vi "Kalman_Estimator_Sepios.vi"(8 "error in":errorcluster) -> (0 "error out":errorcluster)   [LabVIEW 2013]
uses:
  Controls/EKF_Settings.ctl
  Controls/Estimated Position.ctl
  myRIO/Sensors/IMU/IMU_Data_Type_Def.ctl
  <vilib>/imath/engines/lvmath2/RunTimeEngine/ErrorHandling/NIMS_Finalize Error.vi
  <vilib>/imath/engines/lvmath2/RunTimeEngine/BuiltInFunctions/transpose/NIMS_transpose(GV).vi
  <instcachedir>/0/NIMS_transpose(GV)_1D76875BF542458FA31D2D0CC3E998C0.lvgen/NIMS_transpose(GV)_1D76875BF542458FA31D2D0CC3E998C0_000.vi
  <vilib>/imath/engines/lvmath2/RunTimeEngine/NodeEndStatement/NIMS_NodeEndStatement_Output.vi
  <instcachedir>/0/NIMS_NodeEndStatement_Output_53EC0D466D134D7ABD903AC30B43404B.lvgen/NIMS_NodeEndStatement_Output_53EC0D466D134D7ABD903AC30B43404B_003.vi
  <vilib>/imath/engines/lvmath2/RunTimeEngine/IndexRead/NIMS M(R2,S).vi
  <instcachedir>/0/NIMS M(R2,S)_56813DCFDD5A484292D2195AF15D2BF5.lvgen/NIMS M(R2,S)_56813DCFDD5A484292D2195AF15D2BF5_000.vi
  LabVIEW Data/MathScriptVIs/MCStatic_31886544032_2b8e9d258c2bd0716154cc05b7ba0fc2.vi
  <instcachedir>/0/MCStatic_31886544032_2b8e9d258c2bd0716154cc05b7ba0fc2_7C617B4E47594FCE907F90DAAB7145D8.lvgen/MCStatic_31886544032_2b8e9d258c2bd0716154cc05b7ba0fc2_7C617B4E47594FCE907F90DAAB7145D8_001.vi
  <vilib>/imathl/engines/lvmath/Functions/Error Handling/Create Error.vi
  <vilib>/Analysis/Matrix/Numeric/Conversions/Array To Matrix - RA.vi
  <vilib>/imath/engines/lvmath2/RunTimeEngine/Managers/WorkSpace/UID Generator.vi
  <vilib>/Analysis/Matrix/Numeric/Conversions/Matrix To Array - RM.vi
  <vilib>/imath/engines/lvmath2/RunTimeEngine/Managers/SymbolTable/Clear UID.vi
  <instcachedir>/0/NIMS_NodeEndStatement_Output_53EC0D466D134D7ABD903AC30B43404B.lvgen/NIMS_NodeEndStatement_Output_53EC0D466D134D7ABD903AC30B43404B_005.vi
  <instcachedir>/0/NIMS_NodeEndStatement_Output_53EC0D466D134D7ABD903AC30B43404B.lvgen/NIMS_NodeEndStatement_Output_53EC0D466D134D7ABD903AC30B43404B_002.vi
  <vilib>/imath/engines/lvmath2/RunTimeEngine/IndexRead/NIMS M($,S).vi
  <instcachedir>/0/NIMS M($,S)_3E5749BBB62E49528D4765A77F1F6D98.lvgen/NIMS M($,S)_3E5749BBB62E49528D4765A77F1F6D98_000.vi
  LabVIEW Data/MathScriptVIs/MCStatic_31886544032_64f10158a8bf12996c49fb21306ba776.vi
  <instcachedir>/0/MCStatic_31886544032_64f10158a8bf12996c49fb21306ba776_B5FBB23362534537B3F8C988888AB429.lvgen/MCStatic_31886544032_64f10158a8bf12996c49fb21306ba776_B5FBB23362534537B3F8C988888AB429_001.vi
  <vilib>/imath/engines/lvmath2/RunTimeEngine/RunTimeType/NIMS_RunTimeType_From StrictType (excl LVString).vi
  <instcachedir>/0/NIMS_RunTimeType_From StrictType (excl LVString)_4DEE718D6EB74582AA20236969C084FC.lvgen/NIMS_RunTimeType_From StrictType (excl LVString)_4DEE718D6EB74582AA20236969C084FC_000.vi
  <vilib>/imath/engines/lvmath2/RunTimeEngine/LocalVariableDefStatement/MC_LocalVariableDefStatement_Display.vi
  <vilib>/imath/engines/lvmath2/RunTimeEngine/ErrorHandling/NIMS_Create Error From Enums.vi
  <instcachedir>/0/MCStatic_31886544032_64f10158a8bf12996c49fb21306ba776_B5FBB23362534537B3F8C988888AB429.lvgen/MCStatic_31886544032_64f10158a8bf12996c49fb21306ba776_B5FBB23362534537B3F8C988888AB429_000.vi
  Kalman_Estimator_Matlab_Sepios/matlab_tools/quaternion/q_q2rpy.m
  Kalman_Estimator_Matlab_Sepios/matlab_tools/kalman_filter/extended_kalman_filter_process_wpressure_offset_compass_exinit.m
  Kalman_Estimator_Matlab_Sepios/matlab_tools/quaternion/q_min.m
  Kalman_Estimator_Matlab_Sepios/matlab_tools/quaternion/q_mul.m
  Kalman_Estimator_Matlab_Sepios/matlab_tools/quaternion/q_norm.m
  Kalman_Estimator_Matlab_Sepios/matlab_tools/quaternion/q_q2R.m
  Kalman_Estimator_Matlab_Sepios/matlab_tools/quaternion/q_w2Omega.m
  Kalman_Estimator_Matlab_Sepios/matlab_tools/quaternion/skewOp.m
  <vilib>/Analysis/Matrix/NI_Matrix.lvlib
  <vilib>/imath/engines/lvmath2/RunTimeEngine/Managers/SymbolTable/NIMS_WorkSpace.lvlib
panel:
  # "quaternion"
  # "p body position"
  # "v body velocity"
  # "gyro bias"
  # "accel bias"
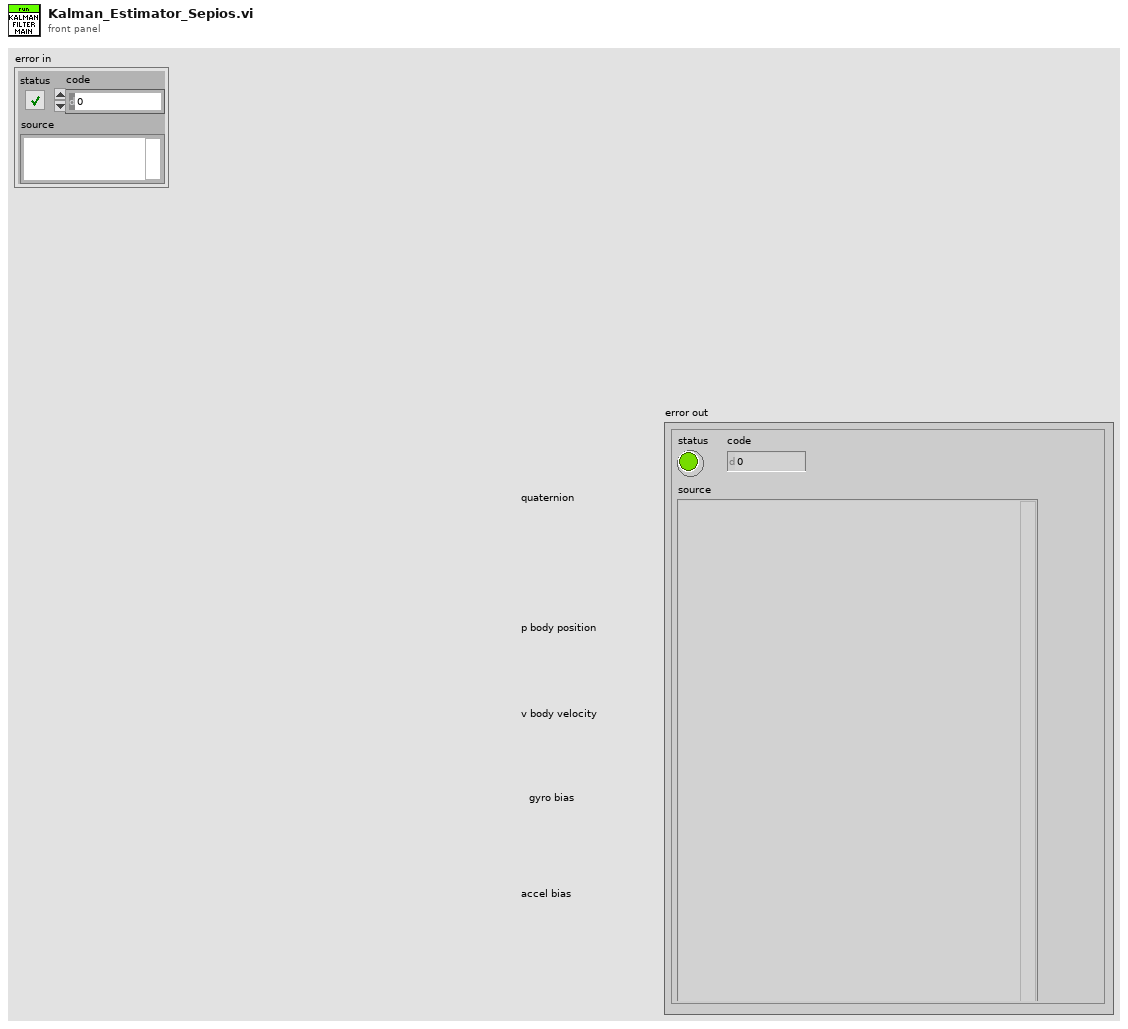
[diagram p1: front panel]
types:
  T1 = typedef "Estimated Position.ctl" = cluster{"X":dbl, "Y":dbl, "Z":dbl, "V_X":dbl, "V_Y":dbl, "V_Z":dbl}
  T2 = typedef "EKF_Settings.ctl" = cluster{"Gravity constant":dbl, "Filter Version":enum16{"IMU Only", "IMU & Pressure", "IMU, Pressure, Compass"}, "Initial Biases":cluster{"Gyro_Bias_nit_x":dbl, "Gyro_Bias_init_y":dbl, "Gyro_Bias_init_z":dbl, "Acc_Bias_init_x":dbl, "Acc_Bias_init_y":dbl, "Acc_Bias_init_z":dbl}, "Use Compass on initialisation":bool, "Initial Biases Covariances":cluster{"Initial_covariance_Gyro_Bias":dbl, "Initial_covariance_Acc_Bias":dbl}, "Magnetic-Field-Vector [utesla]":cluster{"Magf_N_x":dbl, "Magf_N_y":dbl, "Magf_N_z":dbl}, "IMU_Sigmas":cluster{"Sigma_w":dbl, "Sigma_wb":dbl, "Sigma_a":dbl, "Sigma_ab":dbl, "Sigma_m":dbl}, "Measurement Sigmas":cluster{"Sigma_v":dbl, "Sigma_depth":dbl}}
  T3 = typedef "NI_Matrix.lvlib/RealMatrix.ctl" = dbl[][]
  T4 = typedef "IMU_Data_Type_Def.ctl" = cluster{timestamp, "X_Gyro_Out":dbl, "Y_Gyro_Out":dbl, "Z_Gyro_Out":dbl, "X_Accl_Out":dbl, "Y_Accl_Out":dbl, "Z_Accl_Out":dbl, "X_Magn_Out":dbl, "Y_Magn_Out":dbl, "Z_Magn_Out":dbl, "Temp_Out":dbl, "Barom_Out":dbl}
  T5 = enum16{"IMU Only", "IMU & Pressure", "IMU, Pressure, Compass"}
  T6 = cluster{"Magf_N_x":dbl, "Magf_N_y":dbl, "Magf_N_z":dbl}
  T7 = cluster{"Sigma_w":dbl, "Sigma_wb":dbl, "Sigma_a":dbl, "Sigma_ab":dbl, "Sigma_m":dbl}
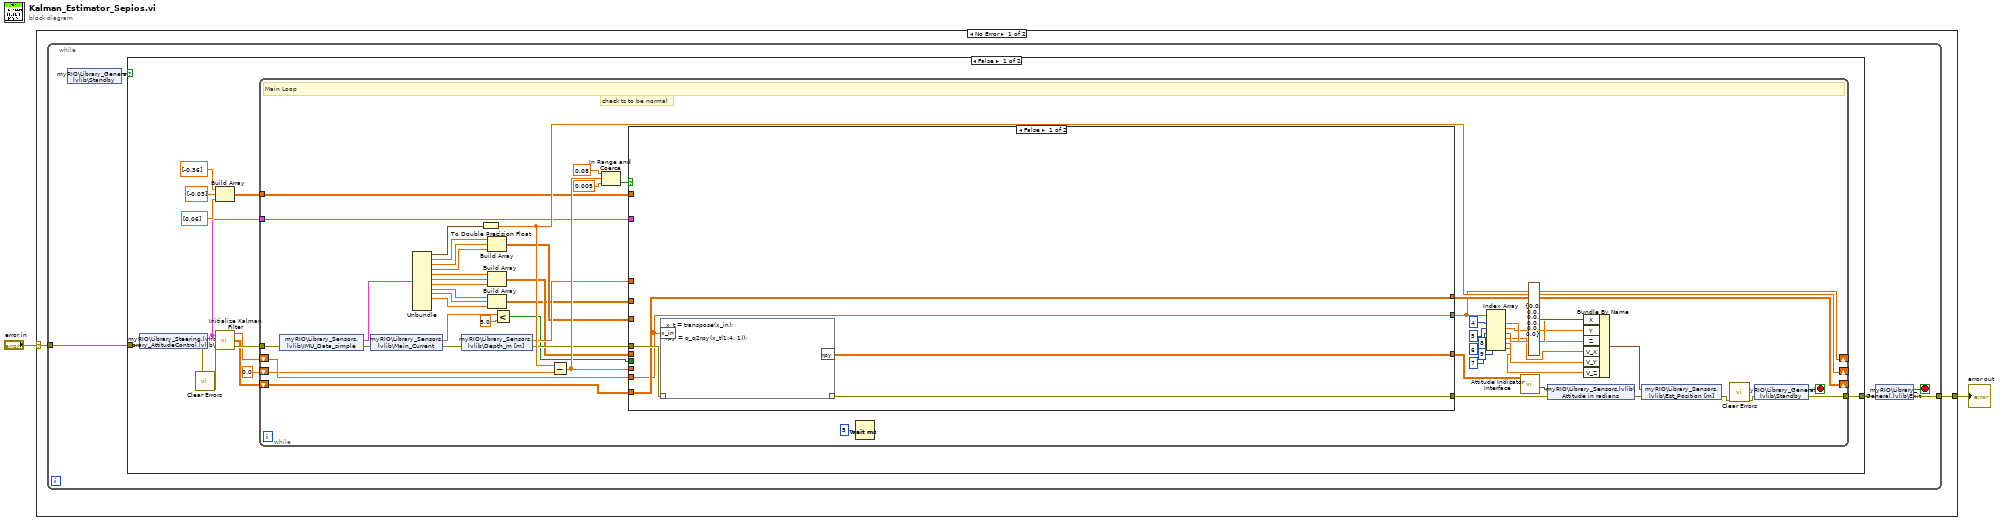
[diagram p0: block diagram]
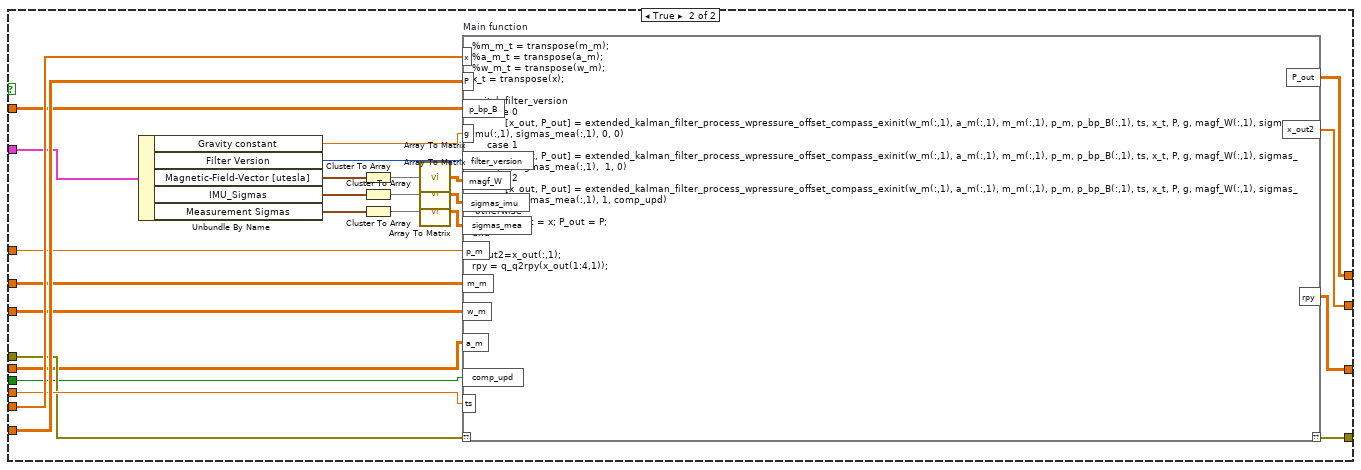
[diagram p2: hidden frame]
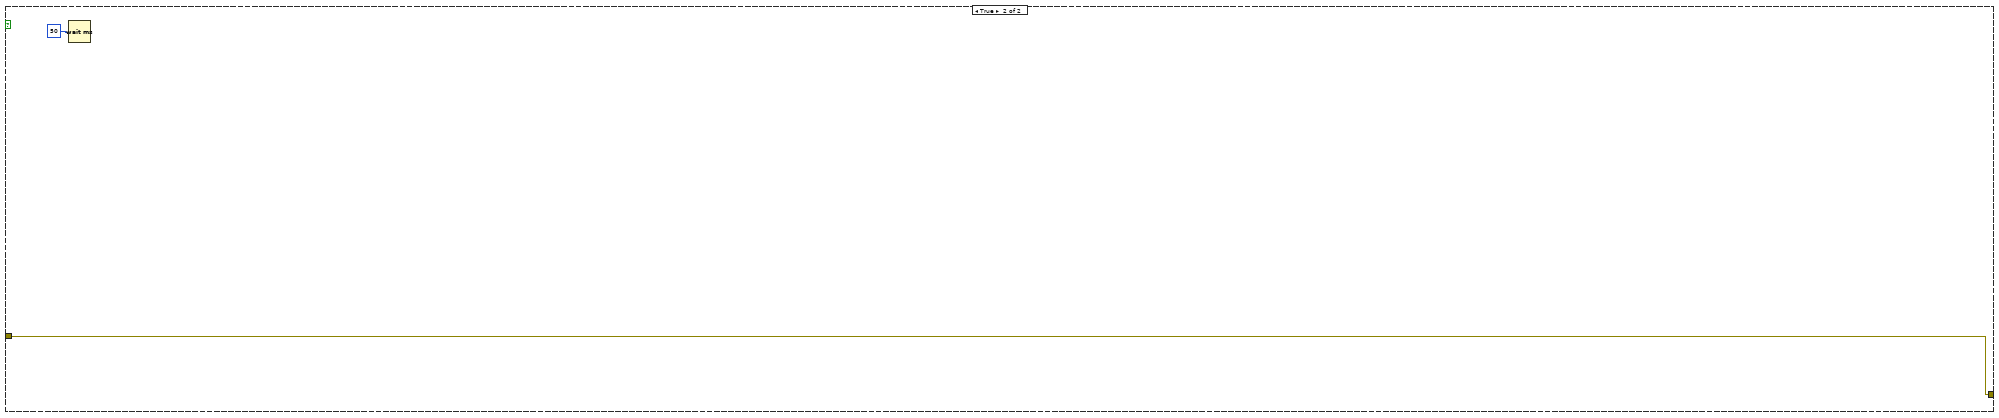
[diagram p3: hidden frame]
diagram:
  n1 = case shown="No Error" "error in" {
    selector: "error in" -> [w3 w646]
    tunnel: [w4 w646] -> w2
    frame No Error {
      n2 = while {
        tunnel: [w5] -> w4
        tunnel: w3 -> [w8]
        stop <- w9 stop-if-true
        n3 = shared-variable "myRIO\\Library_General.lvlib\\Standby"() -> (w7:bool)  [unwired: 1 in, 1 out]
        n4 = case shown="False" w7 {
          tunnel: [w22 w644] -> w6
          tunnel: w8 -> [w18 w644]
          frame False {
            n5 = shared-variable "myRIO\\Library_Steering.lvlib\\Library_AttitudeControl.lvlib\\EKF_Settings"(error in=w18) -> (w11:T2, error out=w16:errorcluster)
            n6 = call <vilib>:"Clear Errors.vi"("error in (no error)"=w16) -> ("error out"=w10:errorcluster)  [unwired: 6 in]
            n7 = Build Array(dbl[] [-0.36] ("element"), dbl[] [-0.03] ("element"), dbl[] [0.06] ("element")) -> (w17:T3)
            n8 = call "Initialize Kalman Filter.vi"("EKF_Settings"=w11, "error in"=w10) -> ("x_init"=w14:dbl[], "P_init"=w13:dbl[][], "error Out"=w15:errorcluster)
            n9 = while {
              tunnel: [w70] -> w22
              shift-right: [w36] -> _
              shift-left: w13 -> [w79]
              shift-right: [w35] -> _
              shift-left: w14 -> [w78]
              tunnel: w15 -> [w72]
              shift-right: [w76] -> _
              shift-left: 0.0 -> [w75]
              tunnel: w17 -> [w62]
              tunnel: w11 -> [w42]
              stop <- w71 stop-if-true
              # "check ts to be normal"
              # "Main Loop"
              n10 = shared-variable "myRIO\\Library_Sensors.lvlib\\IMU_Data_simple"(error in=w72) -> (w74:T4, error out=w54:errorcluster)
              n11 = shared-variable "myRIO\\Library_Sensors.lvlib\\Main_Current"(error in=w54) -> (w51:dbl, error out=w53:errorcluster)
              n12 = Unbundle(w74) -> (w77:timestamp, "X_Gyro_Out"=w50:dbl, "Y_Gyro_Out"=w49:dbl, "Z_Gyro_Out"=w48:dbl, "X_Accl_Out"=w47:dbl, "Y_Accl_Out"=w46:dbl, "Z_Accl_Out"=w45:dbl, "X_Magn_Out"=w34:dbl, "Y_Magn_Out"=w32:dbl, "Z_Magn_Out"=w33:dbl)  [unwired: 2 out]
              n13 = shared-variable "myRIO\\Library_Sensors.lvlib\\Depth_m [m]"(error in=w53) -> (w61:dbl, error out=w52:errorcluster)
              n14 = To Double Precision Float(number=w77) -> (double precision float=w76:dbl)
              n15 = Build Array(w50, w49, w48) -> (w44:T3)
              n16 = Build Array(w47, w46, w45) -> (w43:T3)
              n17 = Build Array(w34, w32, w33) -> (w31:T3)
              n18 = Less?(x=w51, y=5.0) -> (x < y?=w41:bool)
              n19 = Subtract(x=w76, y=w75) -> (x-y=w64:dbl)
              n20 = In Range and Coerce(upper limit=0.08 ("y"), x=w64, lower limit=0.005 ("y")) -> (In Range?=w63:bool)  [unwired: 1 out]
              n21 = case shown="False" w63 {
                tunnel: w79 -> [w81 w158]
                tunnel: [w81 w157] -> w36
                tunnel: w78 -> [w80 w156]
                tunnel: w64 -> [_ w155]
                tunnel: [w84 w154] -> w73
                tunnel: w52 -> [w83 w153]
                tunnel: [w82 w152] -> w68
                tunnel: w62 -> [_ w151]
                tunnel: w61 -> [_ w150]
                tunnel: w41 -> [_ w149]
                tunnel: w44 -> [_ w148]
                tunnel: w43 -> [_ w147]
                tunnel: w42 -> [_ w146]
                tunnel: [w80 w134] -> w35
                tunnel: w31 -> [_ w133]
                frame False {
                  n22 = mathscript code="x_t = transpose(x_in);\n\nrpy = q_q2rpy(x_t(1:4, 1));"("??"=w83, "x_in"=w80) -> ("??"=w82:errorcluster, "rpy"=w84:cdb[][])
                }
                frame True {
                  n23 = Unbundle By Name(w146) -> ("Gravity constant"=w145:dbl, "Filter Version"=w144:T5, "Magnetic-Field-Vector [utesla]"=w143:T6, "IMU_Sigmas"=w138:T7, "Measurement Sigmas"=w137:cluster{"Sigma_v":dbl, "Sigma_depth":dbl})
                  n24 = Cluster To Array(cluster=w143) -> (array=w142:dbl[])
                  n25 = Cluster To Array(cluster=w138) -> (array=w140:dbl[])
                  n26 = Cluster To Array(cluster=w137) -> (array=w139:dbl[])
                  n27 = call-poly <vilib>:"Array To Matrix.vi"("Real 1D Array"=w142) -> ("Real Matrix (Column Vector)"=w141:T3)
                  n28 = call-poly <vilib>:"Array To Matrix.vi"("Real 1D Array"=w140) -> ("Real Matrix (Column Vector)"=w135:T3)
                  n29 = call-poly <vilib>:"Array To Matrix.vi"("Real 1D Array"=w139) -> ("Real Matrix (Column Vector)"=w136:T3)
                  n30 = mathscript code="%m_m_t = transpose(m_m);\n%a_m_t = transpose(a_m);\n%w_m_t = transpose(w_m);\nx_t = transpose(x);\n\nswitch filter_version\n     case 0\n           [x_out, P_out] = extended_kalman_filter_process_wpressure_offset_compass_exinit(w_m(:,1), a_m(:,1), m_m(:,1), p_m, p_bp_B(:,1), ts, x_t, P, g, magf_W(:,1), sigmas_imu(:,1), sigmas_mea(:,1), 0, 0)\n     case 1\n           [x_out, P_out] = extended_kalman_filter_process_wpressure_offset_compass_exinit(w_m(:,1), a_m(:,1), m_m(:,1), p_m, p_bp_B(:,1), ts, x_t, P, g, magf_W(:,1), sigmas_imu(:,1), sigmas_mea(:,1),  1, 0)\n     case 2 \n           [x_out, P_out] = extended_kalman_filter_process_wpressure_offset_compass_exinit(w_m(:,1), a_m(:,1), m_m(:,1), p_m, p_bp_B(:,1), ts, x_t, P, g, magf_W(:,1), sigmas_imu(:,1), sigmas_mea(:,1), 1, comp_upd)\n otherwise\n            x_out = x; P_out = P;\nend\n\nx_out2=x_out(:,1);\nrpy = q_q2rpy(x_out(1:4,1));" "Main function"("??"=w153, "a_m"=w147, "w_m"=w148, "ts"=w155, "P"=w158, "x"=w156, "p_bp_B"=w151, "filter_version"=w144, "p_m"=w150, "g"=w145, "comp_upd"=w149, "m_m"=w133, "magf_W"=w141, "sigmas_imu"=w135, "sigmas_mea"=w136) -> ("??"=w152:errorcluster, "P_out"=w157:dbl[][], "rpy"=w154:cdb[][], "x_out2"=w134:dbl[])
                }
              }
              n31 = Wait (ms)(milliseconds to wait=u32 5) -> ()  [unwired: 1 out]
              n32 = Index Array(array=w35, index #1=4 ("index"), index #2=5 ("index"), index #3=6 ("index"), index #4=7 ("index"), index #5=8 ("index"), index #6=9 ("index")) -> (element #1=w39:dbl, element #2=w38:dbl, element #3=w37:dbl, element #4=w25:dbl, element #5=w24:dbl, element #6=w23:dbl)
              n33 = call "Attitude Indicator Interface.vi"("RPY-Array"=w73) -> ("Attitude in radians"=w67:cluster{"Roll":dbl, "Pitch":dbl, "Yaw":dbl})  [unwired: 9 in, 1 out]
              n34 = shared-variable "myRIO\\Library_Sensors.lvlib\\Attitude in radians"(w67, error in=w68) -> (error out=w55:errorcluster)
              n35 = Bundle By Name(cluster=T1 {"X"=0.0, "Y"=0.0, "Z"=0.0, "V_X"=0.0, "V_Y"=0.0, "V_Z"=0.0} ("Est_Position [m]"), "X"=w39, "Y"=w38, "Z"=w37, "V_X"=w25, "V_Y"=w24, "V_Z"=w23) -> (w57:T1)
              n36 = shared-variable "myRIO\\Library_Sensors.lvlib\\Est_Position [m]"(w57, error in=w55) -> (error out=w29:errorcluster)
              n37 = call <vilib>:"Clear Errors.vi"("error in (no error)"=w29) -> ("error out"=w30:errorcluster)  [unwired: 6 in]
              n38 = shared-variable "myRIO\\Library_General.lvlib\\Standby"(error in=w30) -> (w71:bool, error out=w70:errorcluster)
            }
          }
          frame True {
            n39 = Wait (ms)(milliseconds to wait=u32 50) -> ()  [unwired: 1 out]
          }
        }
        n40 = shared-variable "myRIO\\Library_General.lvlib\\Exit"(error in=w6) -> (w9:bool, error out=w5:errorcluster)
      }
    }
    frame Error {
    }
  }
  "error out" <- w2
